vi "InitCamera.vi"(9 "format string":string, 10 "Image Size":T2, 11 "refnum name":string) -> (3 "CameraDevRef":T1)   [LabVIEW 2016]
uses:
  <vilib>/Rock Robotics/WPI/Camera/WPI_CameraImageSize.ctl
  <vilib>/Rock Robotics/WPI/Camera/WPI_CameraDevRef.ctl
  <vilib>/Rock Robotics/WPI/Camera/WPI_CameraWhite Balance Values.ctl
  <vilib>/Rock Robotics/WPI/Camera/WPI_CameraExposure Values.ctl
  <vilib>/Rock Robotics/WPI/Camera/WPI_CameraFrameRate.ctl
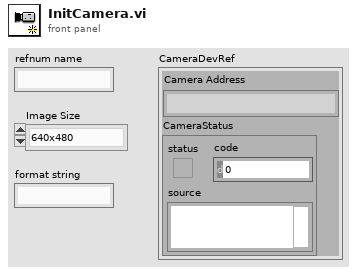
[diagram p1: front panel]
types:
  T1 = typedef "WPI_CameraDevRef.ctl" = cluster{"Camera Address":string, "CameraStatus":errorcluster}
  T2 = typedef "WPI_CameraImageSize.ctl" = enum16{"640x480", "320x240", "160x120", "Custom"}
  T3 = typedef "WPI_CameraFrameRate.ctl" = u32
  T4 = typedef "WPI_CameraExposure Values.ctl" = enum16{"Auto", "Flicker-free 50 Hz", "Flicker-free 60 Hz", "Hold current", "Custom"}
  T5 = typedef "WPI_CameraWhite Balance Values.ctl" = enum16{"Auto", "Fixed indoor", "Fixed outdoor 1", "Fixed outdoor 2", "Fixed fluorescent 1", "Fixed fluorescent 2", "Hold current", "Custom"}
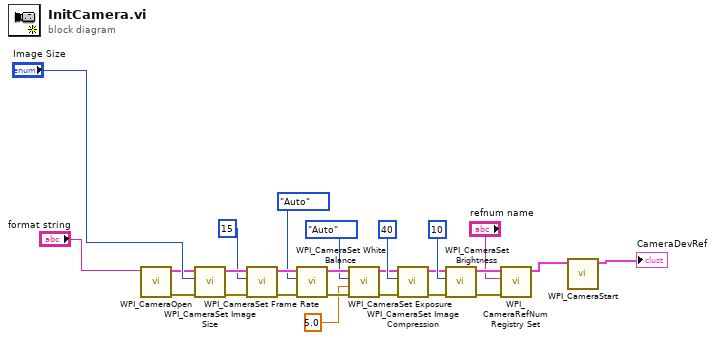
[diagram p0: block diagram]
diagram:
  n1 = call <vilib>:"WPI_CameraOpen.vi"("Camera Address"="format string") -> ("error out"=w13:errorcluster, "CameraDevRef"=w14:T1)  [unwired: 1 in, 8 out]
  n2 = call <vilib>:"WPI_CameraSet Image Size.vi"("error in (no error)"=w13, "Image Size"="Image Size", "CameraDevRef"=w14) -> ("error out"=w12:errorcluster, "CameraDevRef Out"=w15:T1)  [unwired: 1 in, 6 out]
  n3 = call <vilib>:"WPI_CameraSet Frame Rate.vi"("error in (no error)"=w12, "Frame Rate (fps)"=T3 15, "CameraDevRef"=w15) -> ("error out"=w11:errorcluster, "CameraDevRef Out"=w17:T1)  [unwired: 7 out]
  n4 = call <vilib>:"WPI_CameraSet White Balance.vi"("error in (no error)"=w11, "White Balance"=WPI_CameraWhite_Balance_Values."Auto", "CameraDevRef"=w17) -> ("error out"=w10:errorcluster, "CameraDevRef Out"=w16:T1)  [unwired: 1 in, 6 out]
  n5 = call <vilib>:"WPI_CameraSet Exposure.vi"("error in (no error)"=w10, "Exposure (%)"=5.0, "Exposure"=WPI_CameraExposure_Values."Auto", "CameraDevRef"=w16) -> ("error out"=w9:errorcluster, "CameraDevRef Out"=w19:T1)  [unwired: 6 out]
  n6 = call <vilib>:"WPI_CameraSet Image Compression.vi"("error in (no error)"=w9, "Compression"=40, "CameraDevRef"=w19) -> ("error out"=w8:errorcluster, "CameraDevRef Out"=w18:T1)  [unwired: 7 out]
  n7 = call <vilib>:"WPI_CameraSet Brightness.vi"("error in (no error)"=w8, "Brightness"=10, "CameraDevRef"=w18) -> ("error out"=w7:errorcluster, "CameraDevRef Out"=w23:T1)  [unwired: 7 out]
  n8 = call <vilib>:"WPI_CameraRefNum Registry Set.vi"("error in (no error)"=w7, "refnum name"="refnum name", "CameraDevRef"=w23) -> ("CameraDevRef"=w2:T1)  [unwired: 1 in, 7 out]
  n9 = call <vilib>:"WPI_CameraStart.vi"("CameraDevRef"=w2) -> ("CameraDevRef"=→"CameraDevRef":T1)  [unwired: 9 in, 1 out]
